vi "Connect -- subVI.vi"(8 "error in (no error)":errorcluster, 11 "VISA Refnum in":refnum<visa-resource-name>) -> (0 "error out":errorcluster, 2 "Connected?":bool, 3 "VISA Refnum out":refnum<visa-resource-name>)   [LabVIEW 2020, in "Lock-in amplifier.lvlib"]
uses:
  Lock-in amplifier.lvlib
  <instrlib>/Stanford Research 830/Stanford Research 830.lvlib
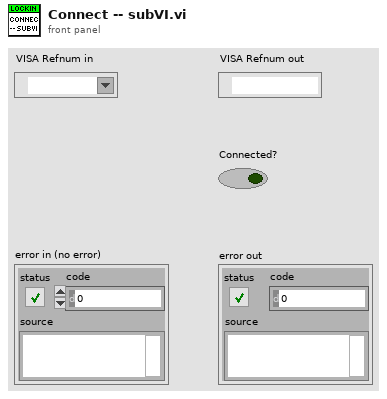
[diagram p1: front panel]
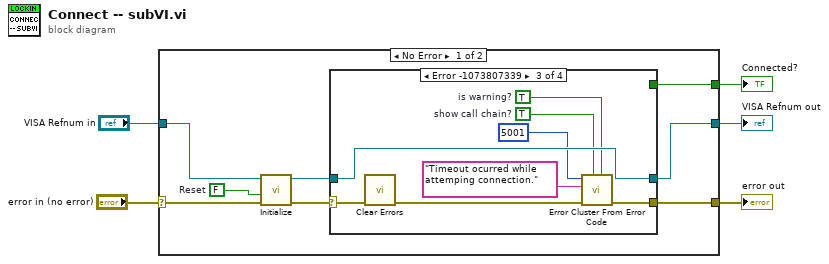
[diagram p0: block diagram]
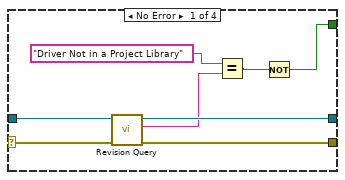
[diagram p2: hidden frame]
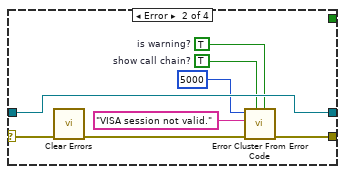
[diagram p3: hidden frame]
diagram:
  n1 = case shown="No Error" "error in (no error)" {
    selector: "error in (no error)" -> [w7 w41]
    tunnel: [w13 w40] -> w5
    tunnel: [w6 _] -> w4
    tunnel: [w12 w41] -> w3
    tunnel: "VISA Refnum in" -> [w8 w40]
    frame No Error {
      w9 = FALSE  # Reset
      n2 = call <instrlib>:"Initialize.vi"("error in (no error)"=w7, "Reset (True)"=w9, "VISA resource name"=w8) -> ("error out"=w11:errorcluster, "VISA resource name out"=w10:refnum<visa-resource-name>)  [unwired: 7 in]
      n3 = case shown="Error -1073807339" w11 {
        selector: w11 -> [w19 w28 w36 w38]
        tunnel: [w21 w29 w37 w39] -> w13
        tunnel: [w20 w26 w34 w38] -> w12
        tunnel: w10 -> [w18 w29 w37 w39]
        tunnel: [w14 _ _ _] -> w6
        frame No Error {
          n4 = call <instrlib>:"Revision Query.vi"("error in (no error)"=w19, "VISA resource name"=w18) -> ("error out"=w20:errorcluster, "Instrument Driver Revision"=w16:string, "VISA resource name out"=w21:refnum<visa-resource-name>)  [unwired: 6 in, 1 out]
          n5 = Equal?(x="Driver Not in a Project Library", y=w16) -> (x = y?=w15:bool)
          n6 = Not(x=w15) -> (.not. x?=w14:bool)
        }
        frame Error {
          w22 = TRUE  # show call chain?
          w24 = TRUE  # is warning?
          n7 = call <vilib>:"Clear Errors.vi"("error in (no error)"=w28) -> ("error out"=w27:errorcluster)  [unwired: 5 in, 1 out]
          n8 = call <vilib>:"Error Cluster From Error Code.vi"("is warning? (False)"=w24, "show call chain? (False)"=w22, "error in (no error)"=w27, "error message (\"\")"="VISA session not valid." ("error message (\"\")"), "error code (0)"=5000) -> ("error out"=w26:errorcluster)  [unwired: 4 in]
        }
        frame Error {
          w30 = TRUE  # show call chain?
          w32 = TRUE  # is warning?
          n9 = call <vilib>:"Clear Errors.vi"("error in (no error)"=w36) -> ("error out"=w35:errorcluster)  [unwired: 5 in, 1 out]
          n10 = call <vilib>:"Error Cluster From Error Code.vi"("is warning? (False)"=w32, "show call chain? (False)"=w30, "error in (no error)"=w35, "error message (\"\")"="Timeout ocurred while attemping connection." ("error message (\"\")"), "error code (0)"=5001) -> ("error out"=w34:errorcluster)  [unwired: 4 in]
        }
        frame Default {
        }
      }
    }
    frame Error {
    }
  }
  "VISA Refnum out" <- w5
  "Connected?" <- w4
  "error out" <- w3
